vi "HumanDriveButtonBoxLeftRight.vi"(8 "DriverBoxRight":bool, 11 "DriverBoxLeft":bool) -> ()   [LabVIEW 2023]
uses:
  HumanGlobal.vi
  <vilib>/Rock Robotics/WPI/ThirdParty/JAS_Junk/TrajLib/Trajectory_Library.lvlib
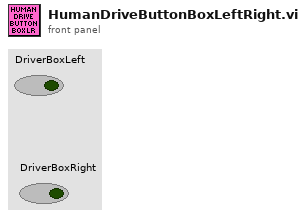
[diagram p1: front panel]
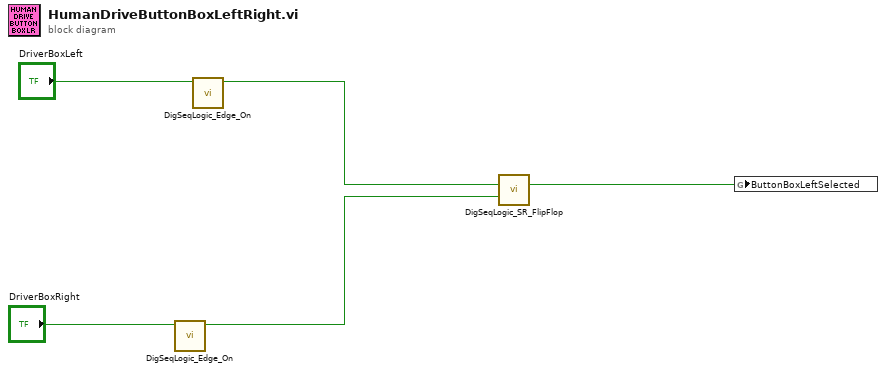
[diagram p0: block diagram]
diagram:
  n1 = call <vilib>:"DigSeqLogic_Edge_On.vi"("Input"="DriverBoxRight") -> ("On Edge"=w2:bool)  [unwired: 10 in]
  n2 = call <vilib>:"DigSeqLogic_Edge_On.vi"("Input"="DriverBoxLeft") -> ("On Edge"=w3:bool)  [unwired: 10 in]
  n3 = call <vilib>:"DigSeqLogic_SR_FlipFlop.vi"("Set"=w3, "Reset"=w2) -> ("Output"=w1:bool)  [unwired: 12 in, 1 out]
  n4 = global write "HumanGlobal.vi" "ButtonBoxLeftSelected"(w1) -> ()
